vi "N_to_Nm.vi"(11 "Force [N]":dbl) -> (3 "Torque [Nm]":dbl)   [LabVIEW 2019]
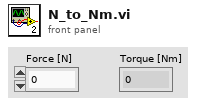
[diagram p1: front panel]
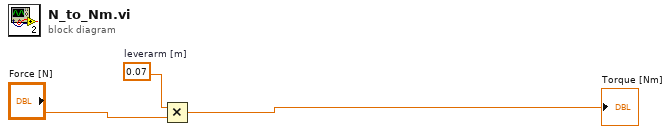
[diagram p0: block diagram]
diagram:
  w1 = 0.07  # leverarm [m]
  n1 = Multiply(x=w1, y="Force [N]") -> (x*y=→"Torque [Nm]":dbl)
